vi "Magnetic Sweep 1.8.vi"() -> ()   [LabVIEW 2011]
uses:
  <vilib>/Math Plots/3D Math Plots/3D Scatter/3D Scatter XCtrl/3D Scatter.xctl
  <vilib>/Math Plots/3D Math Plots/3D Scatter/3D Scatter Datatype/Public/Plot Helper (Vector).vi
  <vilib>/Math Plots/3D Math Plots/3D Scatter/3D Scatter Datatype/3D Scatter Datatype.lvclass
panel:
  out "error out":errorcluster
  in  "error in (no error) 2":errorcluster
  out "x .and. y?":bool
  in  "Initial Temperature":dbl
  out "3D Scatter\n(ramp up)":refnum<class "3D Plot Datatype.lvclass">[](xcontrol)
  out "3D Scatter\n(ramp down)":refnum<class "3D Plot Datatype.lvclass">[](xcontrol)
  out "Heater":bool
  out "Persistent switch ready":bool
  out "error out 6":errorcluster
  in  "Temperature\nlower limite":dbl
  out "Ramping rate command":string
  out "Target field command":string
  out "String":string="Persistent switch is not on"
  in  "Set parameter":bool
  out "status":string
  out "PID command":string
  out "setpoint command":string
  out "setpoint":dbl
  in  "stop":bool
  out "error out 3":errorcluster
  out "error out 2":errorcluster
  in  "Contour plot (ramp down)":path
  in  "Raw data (ramp down)":path
  out "Elapsed Time (s)":dbl
  out "Iteration":i32
  out "Zero field reached":bool
  out "Target field reached":bool
  in  "Temperature\nupper limite":dbl
  in  "Temperature\nramping step":dbl
  in  "Heater range":i16(ring) items=["High", "Medium", "Low"]
  in  "D gain":dbl
  in  "I gain":dbl
  in  "P gain":dbl
  in  "Contour plot (ramp up)":path
  in  "Timer":bool caption="Reset"
  in  "date format":enum16{"short", "long", "abbreviated"}(ring)
  in  "Save":bool
  in  "Raw data (ramp  up)":path
  out "Temperature vs Time":cluster{dbl[], dbl[]}(graph)
  out "current time":timestamp format="%<%I:%M:%S %p\n%x>T"
  out "Magnetic\nField":cluster{dbl[], dbl[]}(graph)
  out "Current Resistance":string
  out "Current Temperature":string
  out "Current Field":string
  out "Status":string
  in  "Field Sweep":bool
  in  "Magnetic field\nRamp rate":dbl
  in  "Traget Field":dbl
  out "Init Response":string
  in  "error in (no error)":errorcluster
  in  "IP Address":string
  in  "Update":bool
  in  "P Switch":bool
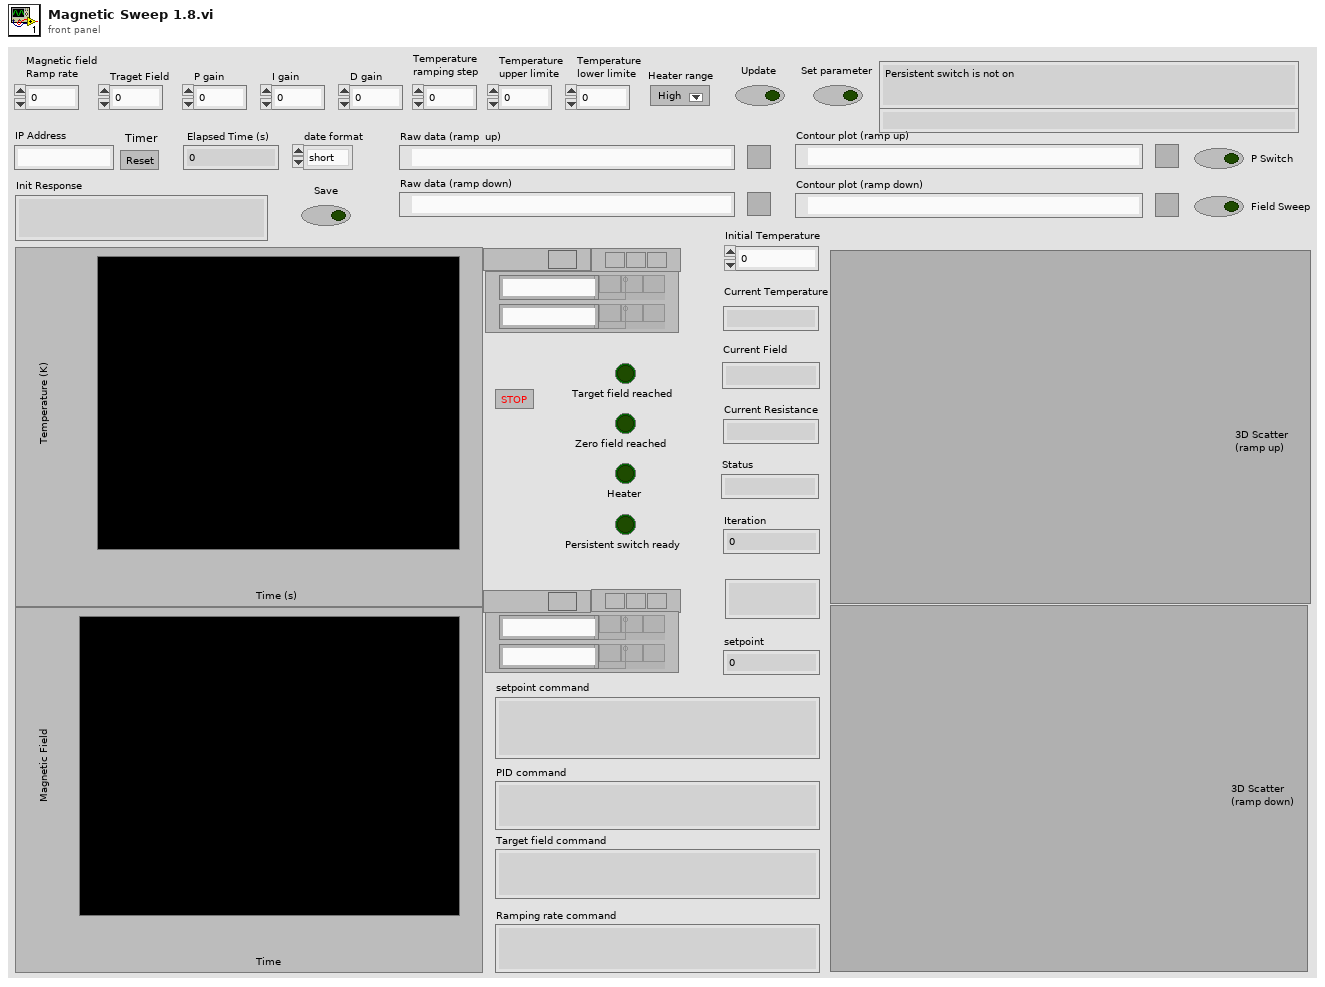
[diagram p1: front panel]
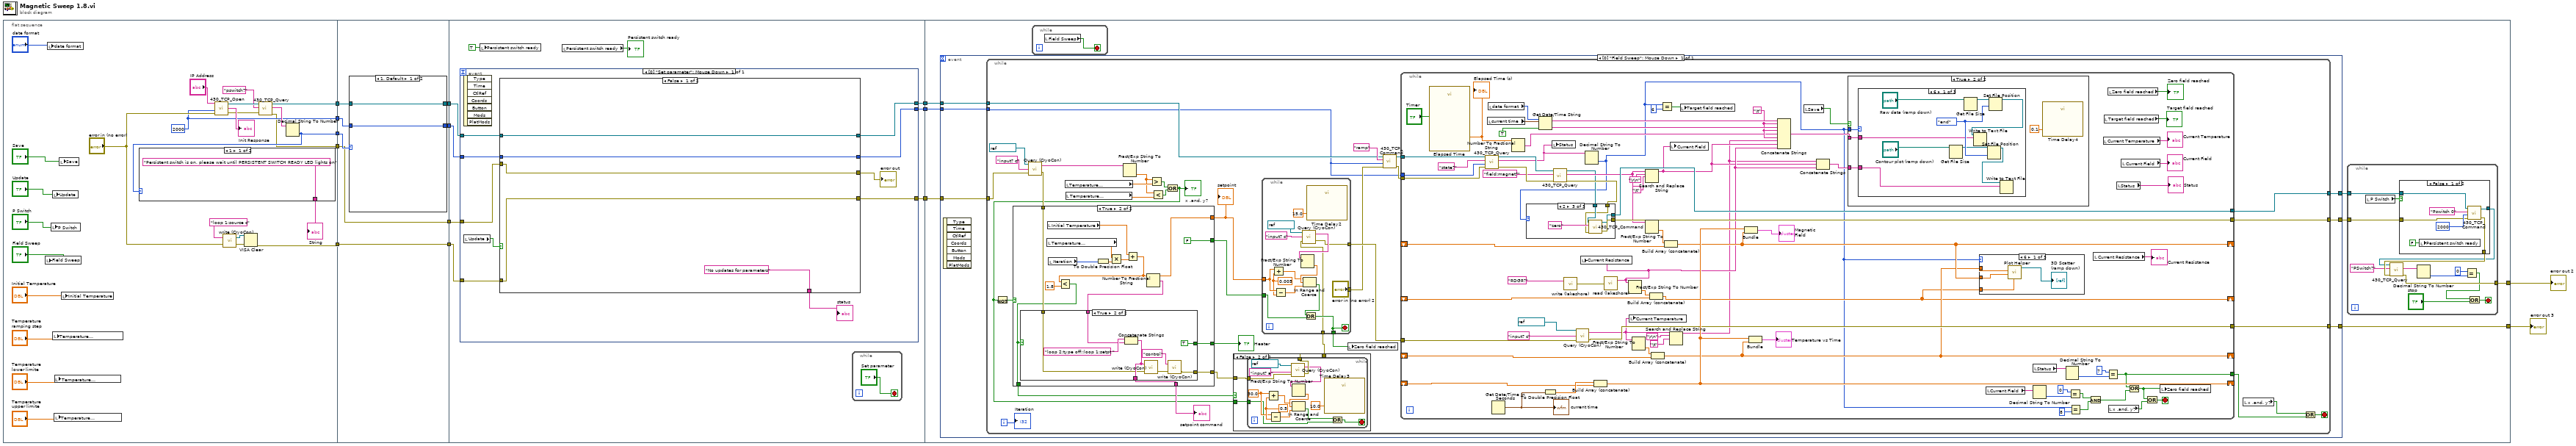
[diagram p0: block diagram]
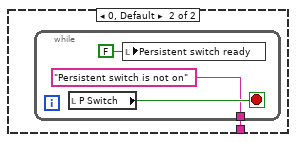
[diagram p2: hidden frame]
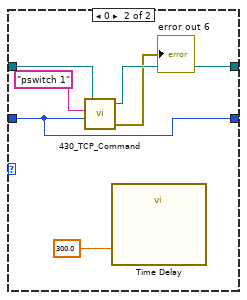
[diagram p3: hidden frame]
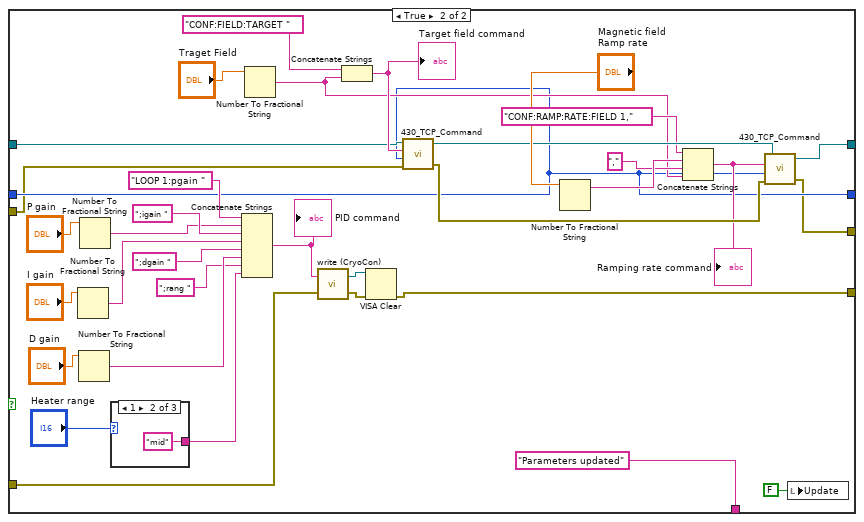
[diagram p4: hidden frame]
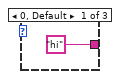
[diagram p5: hidden frame]
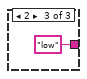
[diagram p6: hidden frame]
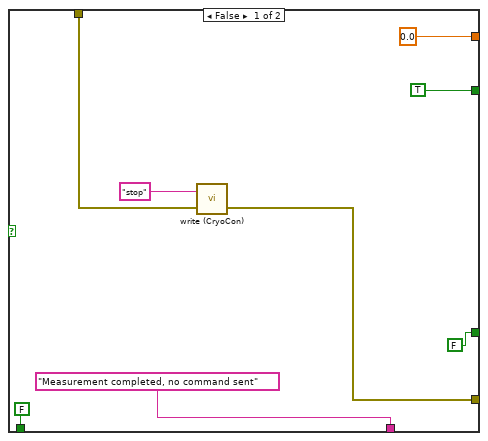
[diagram p9: hidden frame]
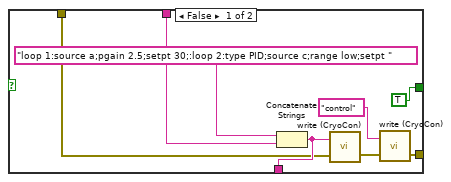
[diagram p10: hidden frame]
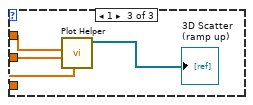
[diagram p12: hidden frame]
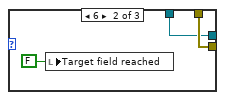
[diagram p14: hidden frame]
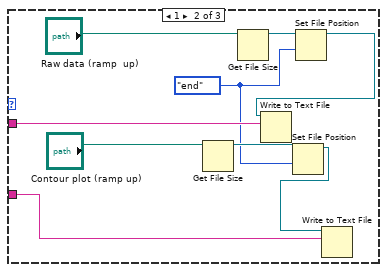
[diagram p16: hidden frame]
diagram:
  n1 = flat-sequence {
    tunnel: [w19] -> w11
    tunnel: [w21] -> w9
    tunnel: [w23] -> w7
    tunnel: [w18] -> w5
    tunnel: [w15] -> w1
    tunnel: w11 -> [w50]
    tunnel: [w48] -> w10
    tunnel: w9 -> [w49]
    tunnel: [w46] -> w8
    tunnel: w7 -> [w51]
    tunnel: [w51] -> w6
    tunnel: w5 -> [w47]
    tunnel: [w45] -> w2
    tunnel: w1 -> [w45]
    tunnel: w10 -> [w61]
    tunnel: w8 -> [w68]
    tunnel: w6 -> [w67]
    tunnel: [w66] -> w14
    tunnel: [w65] -> w13
    tunnel: [w64] -> w12
    tunnel: w2 -> [w60]
    tunnel: w14 -> [w129]
    tunnel: w13 -> [w126]
    tunnel: w12 -> [w125]
    tunnel: [w124] -> w4
    tunnel: [w123] -> w3
    frame #0 {
      w21 = 2000 ("Timeout")
      n2 = local write "Field Sweep"("Field Sweep") -> ()
      n3 = local write "date format"("date format") -> ()
      n4 = local write "P Switch"("P Switch") -> ()
      n5 = local write "Update"("Update") -> ()
      n6 = local write "Temperature\nramping step"("Temperature\nramping step") -> ()
      n7 = local write "Temperature\nupper limite"("Temperature\nupper limite") -> ()
      n8 = local write "Temperature\nlower limite"("Temperature\nlower limite") -> ()
      n9 = local write "Save"("Save") -> ()
      n10 = local write "Initial Temperature"("Initial Temperature") -> ()
      n11 = call "430_TCP_Open.vi"("IP Address"="IP Address", "timeout ms (2000)"=w21, "error in (no error)"="error in (no error)") -> ("connection ID"=w29:refnum<k5>, "Init Response"=→"Init Response":string, "error out"=w28:errorcluster)  [unwired: 3 in]
      n12 = call "write (CryoCon).vi"("error in (no error)"="error in (no error)", "write buffer"="loop 1:source c") -> ("error out"=w25:errorcluster, "VISA resource name out"=w24:refnum<visa-resource-name>)
      n13 = VISA Clear(VISA resource name=w24, error in (no error)=w25) -> (error out=w23:errorcluster)  [unwired: 1 out]
      n14 = call "430_TCP_Query.vi"("error in (no error)"=w28, "Command"="pswitch?", "connection ID"=w29) -> ("error out"=w15:errorcluster, "Response"=w26:string, "connection ID out"=w19:refnum<k5>)  [unwired: 4 in, 2 out]
      n15 = Decimal String To Number(string=w26) -> (number=w18:i32)  [unwired: 2 in, 1 out]
      n16 = case shown="1" w18 {
        tunnel: ["Persistent switch is on, please wait until PERSISTENT SWITCH READY LED lights on" w41] -> w22
        frame 1 {
        }
        frame 0, Default {
          n17 = while {
            tunnel: ["Persistent switch is not on"] -> w41
            stop <- w44 stop-if-true
            n18 = local read "P Switch"() -> (w44:bool)
            n19 = local write "Persistent switch ready"(FALSE ("Persistent switch ready")) -> ()
          }
        }
      }
      "String" <- w22
    }
    frame #1 {
      n20 = case shown="1, Default" w47 {
        tunnel: w50 -> [w53 w59]
        tunnel: w49 -> [w52 w54]
        tunnel: [w53 w58] -> w48
        tunnel: [w52 w54] -> w46
        frame 1, Default {
        }
        frame 0 {
          n21 = call "430_TCP_Command.vi"("Timeout"=w54, "Command"="pswitch 1", "connection ID"=w59) -> ("error out"=→"error out 6":errorcluster, "connection ID out"=w58:refnum<k5>)  [unwired: 1 in, 1 out]
          n22 = call "Time Delay"("Delay Time (s)"=300.0) -> ()  [unwired: 10 in, 1 out]
        }
      }
    }
    frame #2 {
      n23 = event shown="[0] \"Set parameter\": Mouse Down" {
        selector: _ -> [_]
        dyn-events: _ -> [_]
        timeout: _ -> [_]
        tunnel: w61 -> [w79]
        tunnel: w68 -> [w78]
        tunnel: w67 -> [w77]
        tunnel: [w76] -> w66
        tunnel: [w75] -> w65
        tunnel: [w74] -> w64
        tunnel: w60 -> [w71]
        event "Set parameter": Mouse Down {
          n24 = event-data() -> ()  [unwired: 1 in, 7 out]
          n25 = local read "Update"() -> (w72:bool)
          n26 = case shown="False" w72 {
            tunnel: w79 -> [w82 w117]
            tunnel: w78 -> [w83 w90]
            tunnel: w77 -> [w81 w96]
            tunnel: [w81 w86] -> w76
            tunnel: ["No updates for parameters" ("String") "Parameters updated" ("String")] -> w73
            tunnel: [w82 w91] -> w75
            tunnel: [w83 w90] -> w74
            tunnel: w71 -> [w80 w87]
            tunnel: [w80 w85] -> w70
            frame False {
            }
            frame True {
              n27 = Number To Fractional String(number="I gain") -> (F-format string=w100:string)  [unwired: 3 in]
              n28 = Number To Fractional String(number="D gain") -> (F-format string=w98:string)  [unwired: 3 in]
              n29 = Number To Fractional String(number="P gain") -> (F-format string=w101:string)  [unwired: 3 in]
              n30 = case shown="1" "Heater range" {
                tunnel: ["hi" "mid" "low"] -> w93
                frame 0, Default {
                }
                frame 1 {
                }
                frame 2 {
                }
              }
              n31 = Concatenate Strings("LOOP 1:pgain " ("write buffer"), w101, ";igain " ("string"), w100, ";dgain " ("string"), w98, ";rang " ("string"), w93) -> (w97:string)
              "PID command" <- w97
              n32 = Number To Fractional String(number="Traget Field") -> (F-format string=w107:string)  [unwired: 3 in]
              n33 = call "write (CryoCon).vi"("error in (no error)"=w96, "write buffer"=w97) -> ("error out"=w89:errorcluster, "VISA resource name out"=w88:refnum<visa-resource-name>)
              n34 = Concatenate Strings("CONF:FIELD:TARGET ", w107) -> (w118:string)
              "Target field command" <- w118
              n35 = VISA Clear(VISA resource name=w88, error in (no error)=w89) -> (error out=w86:errorcluster)  [unwired: 1 out]
              n36 = call "430_TCP_Command.vi"("error in (no error)"=w87, "Timeout"=w90, "Command"=w118, "connection ID"=w117) -> ("error out"=w116:errorcluster, "connection ID out"=w112:refnum<k5>)  [unwired: 1 out]
              n37 = Number To Fractional String(number="Magnetic field\nRamp rate") -> (F-format string=w110:string)  [unwired: 3 in]
              n38 = Concatenate Strings("CONF:RAMP:RATE:FIELD 1," ("string"), w110, "," ("string"), w107) -> (w113:string)
              "Ramping rate command" <- w113
              n39 = call "430_TCP_Command.vi"("error in (no error)"=w116, "Timeout"=w90, "Command"=w113, "connection ID"=w112) -> ("error out"=w85:errorcluster, "connection ID out"=w91:refnum<k5>)  [unwired: 1 out]
              n40 = local write "Update"(FALSE ("Update")) -> ()
            }
          }
          "status" <- w73
          "error out" <- w70
        }
      }
      n41 = local write "Persistent switch ready"(TRUE ("Persistent switch ready")) -> ()
      n42 = local read "Persistent switch ready"() -> (→"Persistent switch ready":bool)
      n43 = while {
        stop <- "Set parameter" stop-if-true
      }
    }
    frame #3 {
      n44 = event shown="[0] \"Field Sweep\": Mouse Down" {
        selector: _ -> [_]
        dyn-events: _ -> [_]
        timeout: _ -> [_]
        tunnel: w129 -> [w158]
        tunnel: [w157] -> w128
        tunnel: [w156] -> w127
        tunnel: w126 -> [w155]
        tunnel: w125 -> [w154]
        tunnel: [w153] -> w124
        event "Field Sweep": Mouse Down {
          n45 = event-data() -> ()  [unwired: 1 in, 7 out]
          n46 = while {
            tunnel: w158 -> [w175]
            tunnel: [w169] -> w157
            tunnel: [w188] -> w156
            tunnel: w155 -> [w187]
            tunnel: w154 -> [w159]
            tunnel: [w170] -> w153
            i -> [w191]
            stop <- w176 stop-if-true
            n47 = call "Query (CryoCon).vi"("error in (no error)"=w175, "write buffer"="input? c", "VISA resource name 2"=refnum<visa-resource-name> "COM3") -> ("error out"=w173:errorcluster, "read buffer"=w185:string)
            n48 = local read "Temperature\nupper limite"() -> (w189:dbl)
            n49 = local read "Temperature\nlower limite"() -> (w182:dbl)
            n50 = Fract/Exp String To Number(string=w185) -> (number=w183:dbl)  [unwired: 3 in, 1 out]
            n51 = Greater?(x=w183, y=w189) -> (0:w180:bool)
            n52 = Less?(x=w183, y=w182) -> (x < y?=w181:bool)
            n53 = Or(x=w180, y=w181) -> (x .or. y?=w160:bool)
            "x .and. y?" <- w160
            n54 = Not(x=w160) -> (.not. x?=w172:bool)
            n55 = case shown="True" w172 {
              tunnel: [w227 w242] -> w162
              tunnel: [0.0 w240] -> w192
              tunnel: ["Measurement completed, no command sent" w243] -> w171
              tunnel: [TRUE FALSE] -> w179
              tunnel: w173 -> [w229 w236]
              tunnel: [FALSE ("Heater") w235] -> w164
              tunnel: [FALSE w234] -> w163
              frame False {
                n56 = call "write (CryoCon).vi"("error in (no error)"=w229, "write buffer"="stop") -> ("error out"=w227:errorcluster)  [unwired: 1 out]
              }
              frame True {
                n57 = local read "Temperature\nramping step"() -> (w245:dbl)
                n58 = local read "Initial Temperature"() -> (w238:dbl)
                n59 = local read "Iteration"() -> (w237:i32)
                n60 = To Double Precision Float(number=w237) -> (double precision float=w244:dbl)
                n61 = Multiply(x=w245, y=w244) -> (x*y=w246:dbl)
                n62 = Add(x=w238, y=w246) -> (x+y=w240:dbl)
                n63 = Less?(x=w240, y=1.8) -> (x < y?=w234:bool)
                n64 = Number To Fractional String(number=w240) -> (F-format string=w247:string)  [unwired: 3 in]
                n65 = case shown="True" w234 {
                  tunnel: w247 -> [w254 w262]
                  tunnel: [w251 w261] -> w243
                  tunnel: [w253 w260] -> w242
                  tunnel: w236 -> [w248 w257]
                  tunnel: [TRUE ("Heater") TRUE ("Heater")] -> w235
                  frame False {
                    n66 = Concatenate Strings("loop 1:source a;pgain 2.5;setpt 30;:loop 2:type PID;source c;range low;setpt " ("write buffer"), w254) -> (w251:string)
                    n67 = call "write (CryoCon).vi"("error in (no error)"=w248, "write buffer"=w251) -> ("error out"=w250:errorcluster)  [unwired: 1 out]
                    n68 = call "write (CryoCon).vi"("error in (no error)"=w250, "write buffer"="control") -> ("error out"=w253:errorcluster)  [unwired: 1 out]
                  }
                  frame True {
                    n69 = Concatenate Strings("loop 2:type off;:loop 1:setpt " ("write buffer"), w262) -> (w261:string)
                    n70 = call "write (CryoCon).vi"("error in (no error)"=w257, "write buffer"=w261) -> ("error out"=w259:errorcluster)  [unwired: 1 out]
                    n71 = call "write (CryoCon).vi"("error in (no error)"=w259, "write buffer"="control") -> ("error out"=w260:errorcluster)  [unwired: 1 out]
                  }
                }
              }
            }
            "setpoint" <- w192
            "setpoint command" <- w171
            "Heater" <- w164
            n72 = case shown="False" w163 {
              tunnel: w162 -> [w193 w196]
              tunnel: [w193 w195] -> w161
              tunnel: w160 -> [_ w194]
              frame True {
              }
              frame False {
                n73 = while {
                  tunnel: w196 -> [w207]
                  tunnel: [w206] -> w195
                  tunnel: w194 -> [w198]
                  stop <- w197 stop-if-true
                  w200 = 30.0 ("x")
                  w201 = 0.5 ("y")
                  n74 = Add(x=w200, y=w201) -> (x+y=w203:dbl)
                  n75 = Subtract(x=w200, y=w201) -> (x-y=w202:dbl)
                  n76 = call "Query (CryoCon).vi"("error in (no error)"=w207, "write buffer"="input? a", "VISA resource name 2"=refnum<visa-resource-name> "COM3") -> ("error out"=w206:errorcluster, "read buffer"=w205:string)
                  n77 = Fract/Exp String To Number(string=w205) -> (number=w204:dbl)  [unwired: 3 in, 1 out]
                  n78 = In Range and Coerce(upper limit=w203, x=w204, lower limit=w202) -> (In Range?=w199:bool)  [unwired: 1 out]
                  n79 = call "Time Delay3"("Delay Time (s)"=10.0) -> ()  [unwired: 10 in, 1 out]
                  n80 = Or(x=w199, y=w198) -> (x .or. y?=w197:bool)
                }
              }
            }
            n81 = while {
              tunnel: w192 -> [w224]
              tunnel: w179 -> [w216]
              tunnel: [w214] -> w167
              tunnel: ["error in (no error) 2"] -> w166
              tunnel: [w212] -> w165
              tunnel: w161 -> [w211]
              stop <- w212 stop-if-true
              w221 = 0.005 ("y")
              n82 = Add(x=w224, y=w221) -> (x+y=w223:dbl)
              n83 = Subtract(x=w224, y=w221) -> (x-y=w222:dbl)
              n84 = call "Query (CryoCon).vi"("error in (no error)"=w211, "write buffer"="input? c", "VISA resource name 2"=refnum<visa-resource-name> "COM3") -> ("error out"=w214:errorcluster, "read buffer"=w218:string)
              n85 = Fract/Exp String To Number(string=w218) -> (number=w225:dbl)  [unwired: 3 in, 1 out]
              n86 = In Range and Coerce(upper limit=w223, x=w225, lower limit=w222) -> (In Range?=w215:bool)  [unwired: 1 out]
              n87 = Or(x=w215, y=w216) -> (x .or. y?=w212:bool)
              n88 = call "Time Delay2"("Delay Time (s)"=15.0) -> ()  [unwired: 10 in, 1 out]
            }
            n89 = local write "Zero field reached"(w165) -> ()
            n90 = call "430_TCP_Command.vi"("error in (no error)"=w166, "Timeout"=w159, "Command"="ramp", "connection ID"=w187) -> ("error out"=w168:errorcluster, "connection ID out"=w178:refnum<k5>)  [unwired: 1 out]
            n91 = while {
              shift-right: [w305] -> _
              shift-left: _ -> [w334]
              shift-right: [w296] -> _
              shift-left: _ -> [w339]
              shift-right: [w295] -> _
              shift-left: _ -> [w336]
              shift-right: [w331] -> _
              shift-left: _ -> [w292]
              tunnel: w178 -> [w322]
              tunnel: [w304] -> w170
              tunnel: [w308] -> w169
              tunnel: [w307] -> w188
              tunnel: [w274] -> w177
              tunnel: w168 -> [w286]
              tunnel: w167 -> [w285]
              tunnel: w159 -> [w281]
              stop <- w283 stop-if-true
              w325 = "\t"
              n92 = call "Elapsed Time"("Reset"="Timer") -> ("Elapsed Time (s)"=w317:dbl)  [unwired: 11 in, 7 out]
              "Elapsed Time (s)" <- w317
              n93 = call "430_TCP_Query.vi"("error in (no error)"=w286, "Timeout"=w281, "Command"="state?", "connection ID"=w322) -> ("error out"=w280:errorcluster, "Response"=w265:string, "connection ID out"=w278:refnum<k5>)  [unwired: 3 in, 2 out]
              n94 = local read "current time"() -> (w323:timestamp)
              n95 = local read "date format"() -> (w319:enum16{"short", "long", "abbreviated"})
              n96 = Get Date/Time In Seconds() -> (seconds since 1Jan1904=w316:timestamp)
              "current time" <- w316
              n97 = Number To Fractional String(number=w317) -> (F-format string=w320:string)  [unwired: 3 in]
              n98 = Get Date/Time String(date format (0)=w319, seconds (now)=w323, want seconds? (F)=TRUE) -> (date string=w327:string, time string=w326:string)
              n99 = To Double Precision Float(number=w316) -> (double precision float=w293:dbl)
              n100 = local write "Status"(w265) -> ()
              n101 = call "430_TCP_Query.vi"("error in (no error)"=w280, "Command"="field:magnet?", "connection ID"=w278) -> ("error out"=w279:errorcluster, "Response"=w276:string, "connection ID out"=w275:refnum<k5>)  [unwired: 4 in, 2 out]
              n102 = call "write (lakeshore).vi"("write buffer"="RDGR?") -> ("error out"=w338:errorcluster)  [unwired: 1 in]
              n103 = call "Query (CryoCon).vi"("error in (no error)"=w285, "write buffer"="input? c", "VISA resource name 2"=refnum<visa-resource-name> "COM3") -> ("error out"=w304:errorcluster, "read buffer"=w301:string)
              n104 = Decimal String To Number(string=w265) -> (number=w264:i32)  [unwired: 2 in, 1 out]
              n105 = case shown="2" w264 {
                tunnel: [w350 w352 w357] -> w307
                tunnel: [w349 w351 w356] -> w308
                tunnel: w279 -> [w350 w352 w354]
                tunnel: w275 -> [w349 w351 w355]
                frame 0, Default {
                }
                frame 6 {
                  n106 = local write "Target field reached"(FALSE ("Target field reached")) -> ()
                }
                frame 2 {
                  n107 = call "430_TCP_Command.vi"("error in (no error)"=w354, "Command"="zero", "connection ID"=w355) -> ("error out"=w357:errorcluster, "connection ID out"=w356:refnum<k5>)  [unwired: 1 in, 1 out]
                }
              }
              n108 = Build Array (concatenate)(w293, w292) -> (w331:dbl[])
              n109 = call "read (lakeshore).vi"("error in (no error)"=w338) -> ("read buffer"=w294:string)  [unwired: 1 out]
              n110 = local write "Current Resistance"(w294) -> ()
              n111 = Fract/Exp String To Number(string=w294) -> (number=w332:dbl)  [unwired: 3 in, 1 out]
              n112 = local write "Current Temperature"(w301) -> ()
              n113 = Fract/Exp String To Number(string=w301) -> (number=w333:dbl)  [unwired: 3 in, 1 out]
              n114 = Search and Replace String(input string=w276, search string="\r\n", replace string="\t") -> (result string=w291:string)  [unwired: 5 in, 3 out]
              n115 = Fract/Exp String To Number(string=w276) -> (number=w335:dbl)  [unwired: 3 in, 1 out]
              n116 = Build Array (concatenate)(w332, w336) -> (w295:dbl[])
              n117 = Build Array (concatenate)(w333, w339) -> (w296:dbl[])
              n118 = Equal?(x=w264, y=6) -> (x = y?=w321:bool)
              n119 = Build Array (concatenate)(w335, w334) -> (w305:dbl[])
              n120 = Search and Replace String(input string=w301, search string="\r\n", replace string="\t") -> (result string=w290:string)  [unwired: 5 in, 3 out]
              n121 = local write "Current Field"(w291) -> ()
              n122 = local write "Target field reached"(w321) -> ()
              n123 = Bundle(w331, w305) -> (→"Magnetic\nField":cluster{dbl[], dbl[]})  [unwired: 1 in]
              n124 = Bundle(w331, w296) -> (→"Temperature vs Time":cluster{dbl[], dbl[]})  [unwired: 1 in]
              n125 = Concatenate Strings(w327, w325, w326, w325, w320, w325, w290, w291, w294) -> (w330:string)
              n126 = local read "Save"() -> (w315:bool)
              n127 = Concatenate Strings(w290, w291, w294) -> (w324:string)
              n128 = case shown="True" w315 {
                tunnel: w330 -> [_ w362]
                tunnel: w324 -> [_ w361]
                tunnel: w264 -> [_ w360]
                frame False {
                }
                frame True {
                  n129 = case shown="6" w360 {
                    tunnel: w362 -> [w364 w380 _]
                    tunnel: w361 -> [w363 w374 _]
                    frame 6 {
                      w370 = enum16{"start", "end", "current"}."end" ("from (0:start)")
                      n130 = Get File Size(file="Contour plot (ramp down)") -> (refnum out=w369:refnum<file>)  [unwired: 1 in, 2 out]
                      n131 = Get File Size(file="Raw data (ramp down)") -> (refnum out=w366:refnum<file>)  [unwired: 1 in, 2 out]
                      n132 = Set File Position(refnum=w369, from (0:start)=w370) -> (refnum out=w371:refnum<file>)  [unwired: 2 in, 1 out]
                      n133 = Set File Position(refnum=w366, from (0:start)=w370) -> (refnum out=w367:refnum<file>)  [unwired: 2 in, 1 out]
                      n134 = Write to Text File(file (use dialog)=w367, text=w364) -> ()  [unwired: 2 in, 3 out]
                      n135 = Write to Text File(file (use dialog)=w371, text=w363) -> ()  [unwired: 2 in, 3 out]
                    }
                    frame 1 {
                      w373 = enum16{"start", "end", "current"}."end" ("from (0:start)")
                      n136 = Get File Size(file="Contour plot (ramp up)") -> (refnum out=w375:refnum<file>)  [unwired: 1 in, 2 out]
                      n137 = Get File Size(file="Raw data (ramp  up)") -> (refnum out=w378:refnum<file>)  [unwired: 1 in, 2 out]
                      n138 = Set File Position(refnum=w375, from (0:start)=w373) -> (refnum out=w372:refnum<file>)  [unwired: 2 in, 1 out]
                      n139 = Set File Position(refnum=w378, from (0:start)=w373) -> (refnum out=w377:refnum<file>)  [unwired: 2 in, 1 out]
                      n140 = Write to Text File(file (use dialog)=w377, text=w380) -> ()  [unwired: 2 in, 3 out]
                      n141 = Write to Text File(file (use dialog)=w372, text=w374) -> ()  [unwired: 2 in, 3 out]
                    }
                    frame Default {
                    }
                  }
                  n142 = call "Time Delay4"("Delay Time (s)"=0.1) -> ()  [unwired: 10 in, 1 out]
                }
              }
              n143 = case shown="6" w264 {
                tunnel: w296 -> [w342 _ w345]
                tunnel: w305 -> [w341 _ w346]
                tunnel: w295 -> [w343 _ w347]
                frame 6 {
                  n144 = call-poly <vilib>:"Plot Helper.vi"("z vector"=w343, "y vector"=w341, "x vector"=w342) -> ("3D Plot lvclass Array out"=→"3D Scatter\n(ramp down)":refnum<class "3D Plot Datatype.lvclass">[])  [unwired: 3 in, 5 out]
                }
                frame 0, Default {
                }
                frame 1 {
                  n145 = call-poly <vilib>:"Plot Helper.vi"("z vector"=w347, "y vector"=w346, "x vector"=w345) -> ("3D Plot lvclass Array out"=→"3D Scatter\n(ramp up)":refnum<class "3D Plot Datatype.lvclass">[])  [unwired: 3 in, 5 out]
                }
              }
              n146 = local read "Current Field"() -> (w270:string)
              n147 = local read "Status"() -> (w268:string)
              n148 = Decimal String To Number(string=w270) -> (number=w271:i32)  [unwired: 2 in, 1 out]
              n149 = Decimal String To Number(string=w268) -> (number=w267:i32)  [unwired: 2 in, 1 out]
              n150 = Equal?(x=0, y=w271) -> (x = y?=w288:bool)
              n151 = Equal?(x=w264, y=8) -> (x = y?=w289:bool)
              n152 = And(x=w288, y=w289) -> (x .and. y?=w287:bool)
              n153 = local read "Current Resistance"() -> (→"Current Resistance":string)
              n154 = local read "Current Temperature"() -> (→"Current Temperature":string)
              n155 = local read "Target field reached"() -> (→"Target field reached":bool)
              n156 = Equal?(x=7, y=w267) -> (x = y?=w274:bool)
              n157 = local read "Zero field reached"() -> (→"Zero field reached":bool)
              n158 = local read "x .and. y?"() -> (w282:bool)
              n159 = local read "Status"() -> (→"Status":string)
              n160 = local read "Current Field"() -> (→"Current Field":string)
              n161 = Or(x=w274, y=w287) -> (x .or. y?=w284:bool)
              n162 = Or(x=w284, y=w282) -> (x .or. y?=w283:bool)
              n163 = local write "Zero field reached"(w284) -> ()
            }
            n164 = local read "x .and. y?"() -> (w174:bool)
            n165 = Or(x=w174, y=w177) -> (x .or. y?=w176:bool)
            "Iteration" <- w191
          }
        }
      }
      n166 = while {
        stop <- w130 stop-if-true
        n167 = local read "Field Sweep"() -> (w130:bool)
      }
      n168 = while {
        tunnel: w128 -> [w143]
        tunnel: w127 -> [w141]
        tunnel: [w136] -> w123
        stop <- w131 stop-if-true
        n169 = local read "P Switch"() -> (w142:bool)
        n170 = case shown="False" w142 {
          tunnel: w143 -> [w149 w152]
          tunnel: w141 -> [w147 w151]
          tunnel: [w145 w151] -> w139
          tunnel: [w144 w152] -> w138
          frame False {
            n171 = local write "Persistent switch ready"(FALSE ("Persistent switch ready")) -> ()
            n172 = call "430_TCP_Command.vi"("error in (no error)"=w147, "Timeout"=2000, "Command"="Pswitch 0", "connection ID"=w149) -> ("error out"=w145:errorcluster, "connection ID out"=w144:refnum<k5>)  [unwired: 1 out]
          }
          frame True {
          }
        }
        n173 = call "430_TCP_Query.vi"("error in (no error)"=w139, "Command"="PSwitch?", "connection ID"=w138) -> ("error out"=w136:errorcluster, "Response"=w135:string)  [unwired: 4 in, 3 out]
        n174 = Decimal String To Number(string=w135) -> (number=w134:i32)  [unwired: 2 in, 1 out]
        n175 = Equal?(x=0, y=w134) -> (x = y?=w132:bool)
        n176 = Or(x=w132, y="stop") -> (x .or. y?=w131:bool)
      }
    }
  }
  "error out 2" <- w3
  "error out 3" <- w4
